vi "Heat Control Parse (SubVI).vi"(10 "Data":string, 11 "Heat Control in":T1) -> (3 "Heat Control out":T1)   [LabVIEW 2023]
uses:
  type defs/Heat Control.ctl
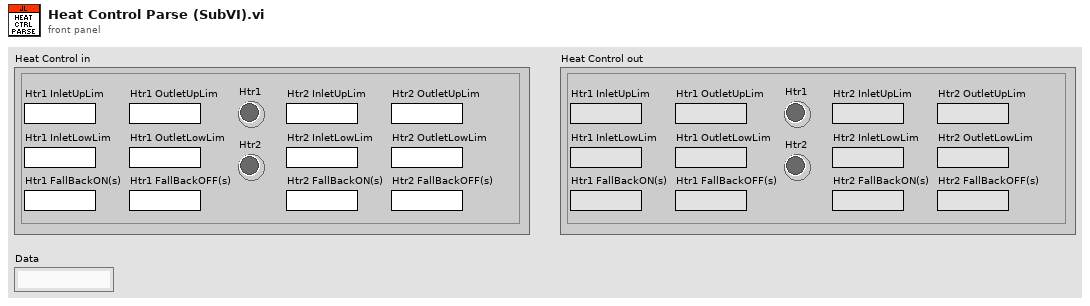
[diagram p1: front panel]
types:
  T1 = typedef "Heat Control.ctl" = cluster{"Htr1 InletLowLim":string, "Htr1 InletUpLim":string, "Htr1 OutletLowLim":string, "Htr1 OutletUpLim":string, "Htr1 FallBackON(s)":string, "Htr1 FallBackOFF(s)":string, "Htr1":bool, "Htr2 InletLowLim":string, "Htr2 InletUpLim":string, "Htr2 OutletLowLim":string, "Htr2 OutletUpLim":string, "Htr2 FallBackON(s)":string, "Htr2 FallBackOFF(s)":string, "Htr2":bool}
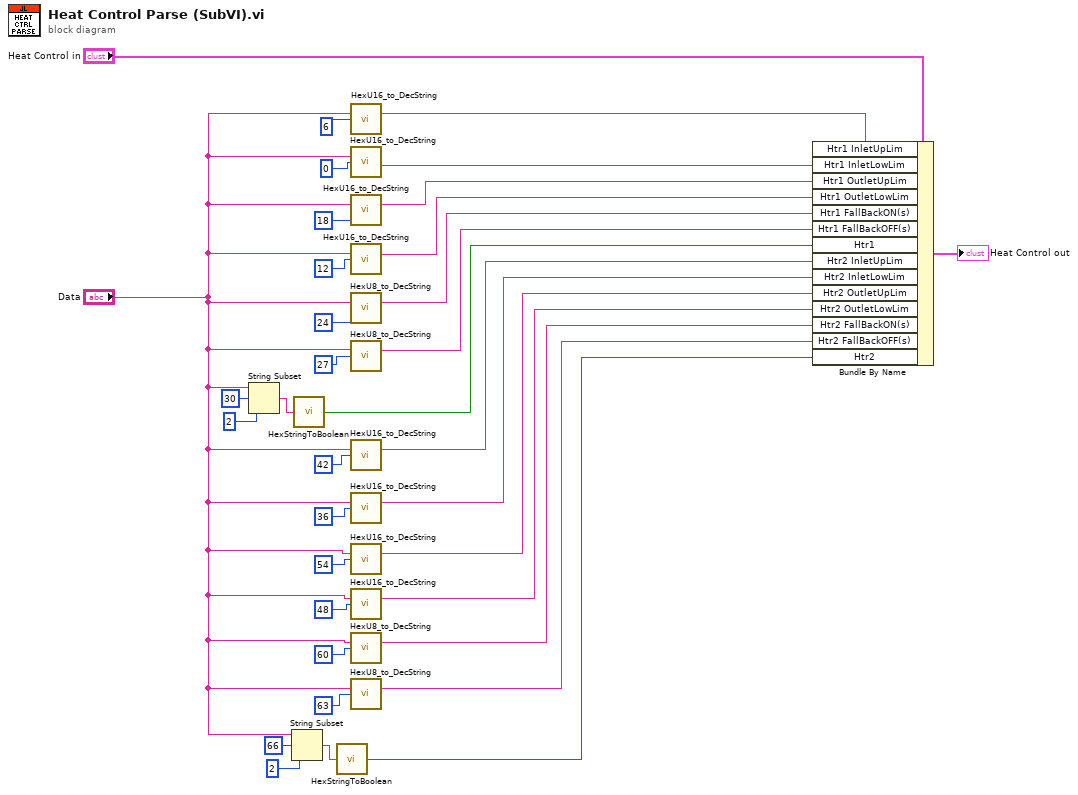
[diagram p0: block diagram]
diagram:
  n1 = String Subset(string="Data", offset (0)=30, length (rest)=2 ("length (rest)")) -> (substring=w34:string)
  n2 = String Subset(string="Data", offset (0)=66, length (rest)=2 ("length (rest)")) -> (substring=w26:string)
  n3 = call "HexStringToBoolean.vi"("Hex String"=w34) -> ("Boolean"=w22:bool)
  n4 = call "HexStringToBoolean.vi"("Hex String"=w26) -> ("Boolean"=w21:bool)
  n5 = call "HexU16_to_DecString.vi"("String"="Data", "offset (0)"=6) -> ("decimal integer string"=w1:string)  [unwired: 12 in, 1 out]
  n6 = call "HexU16_to_DecString.vi"("String"="Data", "offset (0)"=0) -> ("decimal integer string"=w20:string)  [unwired: 12 in, 1 out]
  n7 = call "HexU16_to_DecString.vi"("String"="Data", "offset (0)"=18) -> ("decimal integer string"=w18:string)  [unwired: 12 in, 1 out]
  n8 = call "HexU16_to_DecString.vi"("String"="Data", "offset (0)"=12) -> ("decimal integer string"=w16:string)  [unwired: 12 in, 1 out]
  n9 = call "HexU8_to_DecString.vi"("String"="Data", "offset (0)"=24) -> ("decimal integer string"=w24:string)  [unwired: 13 in]
  n10 = call "HexU8_to_DecString.vi"("String"="Data", "offset (0)"=27) -> ("decimal integer string"=w23:string)  [unwired: 13 in]
  n11 = call "HexU16_to_DecString.vi"("String"="Data", "offset (0)"=42) -> ("decimal integer string"=w14:string)  [unwired: 12 in, 1 out]
  n12 = call "HexU16_to_DecString.vi"("String"="Data", "offset (0)"=36) -> ("decimal integer string"=w13:string)  [unwired: 12 in, 1 out]
  n13 = call "HexU16_to_DecString.vi"("String"="Data", "offset (0)"=54) -> ("decimal integer string"=w12:string)  [unwired: 12 in, 1 out]
  n14 = call "HexU16_to_DecString.vi"("String"="Data", "offset (0)"=48) -> ("decimal integer string"=w11:string)  [unwired: 12 in, 1 out]
  n15 = call "HexU8_to_DecString.vi"("String"="Data", "offset (0)"=60) -> ("decimal integer string"=w10:string)  [unwired: 13 in]
  n16 = call "HexU8_to_DecString.vi"("String"="Data", "offset (0)"=63) -> ("decimal integer string"=w9:string)  [unwired: 13 in]
  n17 = Bundle By Name(cluster="Heat Control in", "Htr1 InletUpLim"=w1, "Htr1 InletLowLim"=w20, "Htr1 OutletUpLim"=w18, "Htr1 OutletLowLim"=w16, "Htr1 FallBackON(s)"=w24, "Htr1 FallBackOFF(s)"=w23, "Htr1"=w22, "Htr2 InletUpLim"=w14, "Htr2 InletLowLim"=w13, "Htr2 OutletUpLim"=w12, "Htr2 OutletLowLim"=w11, "Htr2 FallBackON(s)"=w10, "Htr2 FallBackOFF(s)"=w9, "Htr2"=w21) -> (→"Heat Control out":T1)
